vi "Create Hardware Info.vi"(8 "error in (no error)":errorcluster) -> (0 "error out":errorcluster, 3 "Hardware Info":refnum<class "Hardware Info.lvclass">)   [LabVIEW 2017, in "DSF Core.lvlib" / "Hardware Info.lvclass"]
uses:
  Hardware Info/Hardware Info.lvclass
  Hardware Info/Hardware Info.lvclass/Hardware Info.ctl
  CPU Info/CPU Info.lvclass
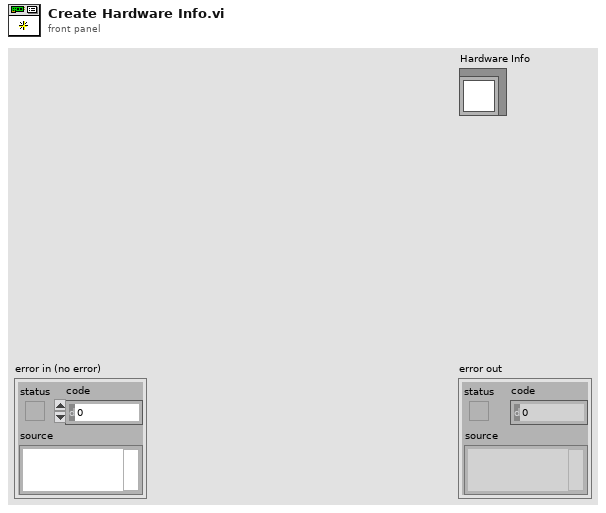
[diagram p1: front panel]
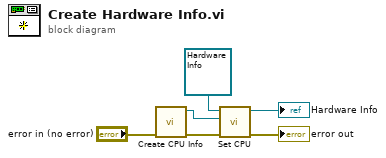
[diagram p0: block diagram]
diagram:
  n1 = call "Create CPU Info.vi"("error in (no error)"="error in (no error)") -> ("error out"=w1:errorcluster, "CPU Info out"=w5:refnum<class "CPU Info.lvclass">)  [unwired: 9 in]
  n2 = call "Set CPU.vi"("error in (no error)"=w1, "CPU Info"=w5, "Hardware Info in"=refnum<class "Hardware Info.lvclass"> refnum) -> ("error out"=→"error out":errorcluster, "Hardware Info out"=→"Hardware Info":refnum<class "Hardware Info.lvclass">)  [unwired: 7 in]
